vi "Calibaration_Correction.vi"(9 "data":dbl[](array[numeric]), 11 "Index Map":i32[](array[numeric])) -> (3 "Calibrated Array":dbl[](array[numeric]))   [LabVIEW 2025]
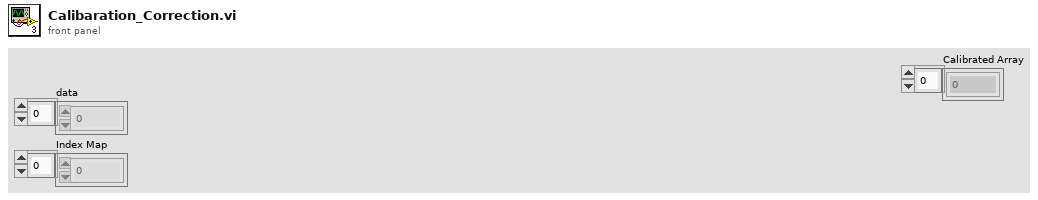
[diagram p1: front panel]
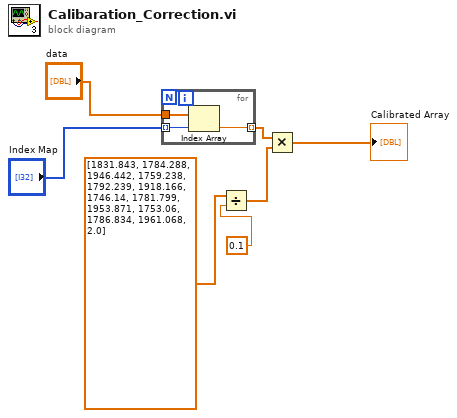
[diagram p0: block diagram]
diagram:
  n1 = for {
    tunnel: "data" -> [w10]
    tunnel: "Index Map" -> [w9] mode=indexing
    tunnel: [w8] -> w4 mode=indexing
    n2 = Index Array(array=w10, index=w9) -> (element=w8:dbl)
  }
  n3 = Divide(x=dbl[] [1831.843, 1784.288, 1946.442, 1759.238, 1792.239, 1918.166, 1746.14, 1781.799, 1953.871, 1753.06, 1786.834, 1961.068, 2.0], y=0.1) -> (x/y=w2:dbl[])
  n4 = Multiply(x=w4, y=w2) -> (x*y=→"Calibrated Array":dbl[])
